vi "UPDATE ITEMS.vi"(10 "DATA IN":T3, 11 "connection reference in":T1) -> (3 "connection reference out":T1)   [LabVIEW 2019]
uses:
  Controls/Table Data Types/Inventory Data Type.ctl
  <vilib>/addons/database/Connection.llb/Conn ObjectReference.ctl
  Controls/Column Names/Inventory Column Names.ctl
  <vilib>/addons/database/NI_Database_API.lvlib
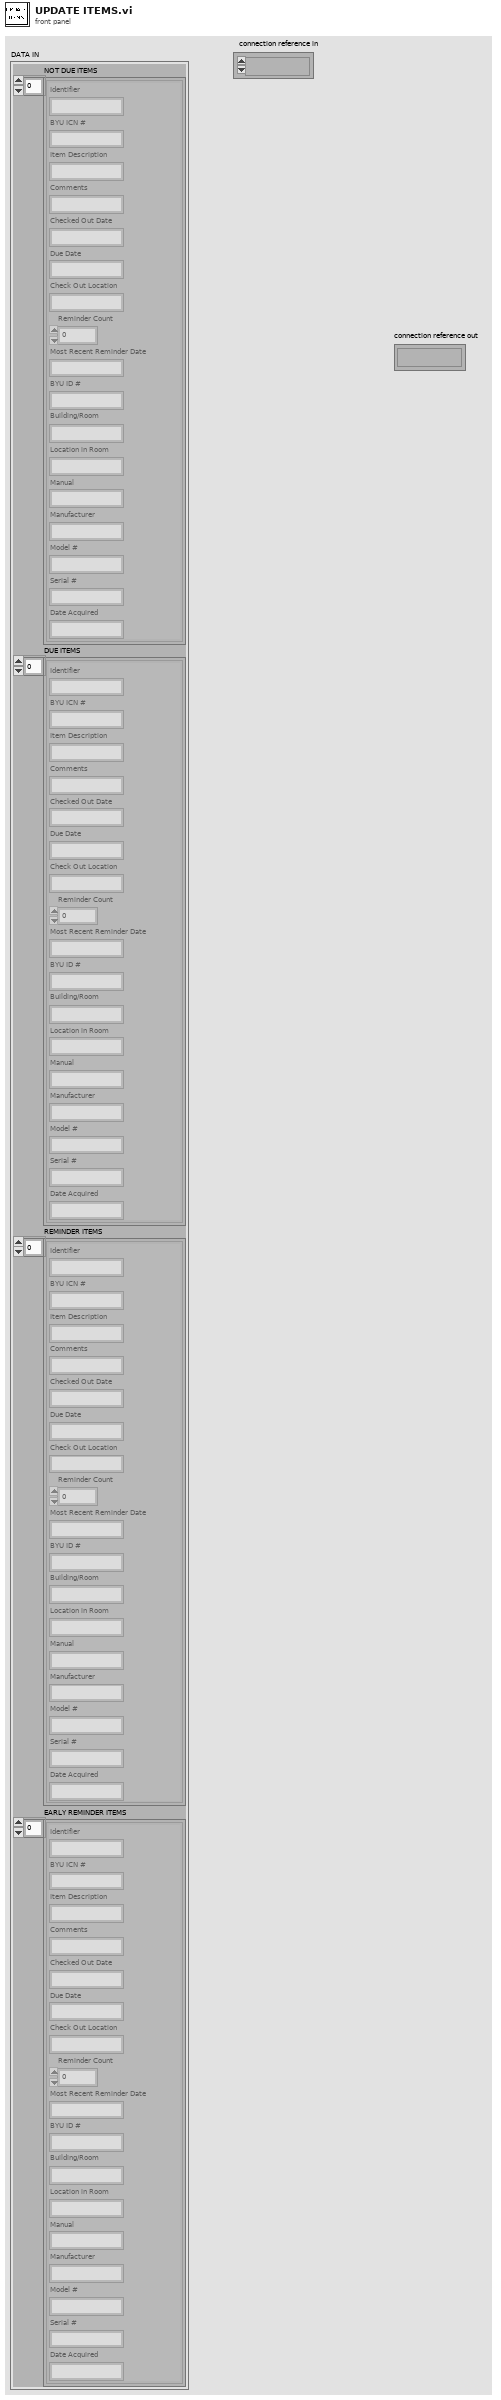
[diagram p1: front panel]
types:
  T1 = typedef "NI_Database_API.lvlib/Conn ObjectReference.ctl" = refnum<k1>
  T2 = typedef "Inventory Data Type.ctl" = cluster{"Identifier":string, "BYU ICN #":string, "Item Description":string, "Comments":string, "Checked Out Date":string, "Due Date":string, "Check Out Location":string, "Reminder Count":i32, "Most Recent Reminder Date":string, "BYU ID #":string, "Building/Room":string, "Location in Room":string, "Manual":string, "Manufacturer":string, "Model #":string, "Serial #":string, "Date Acquired":string}
  T3 = cluster{"NOT DUE ITEMS":T2[], "DUE ITEMS":T2[], "REMINDER ITEMS":T2[], "EARLY REMINDER ITEMS":T2[]}
  T4 = typedef "Inventory Column Names.ctl" = string[]
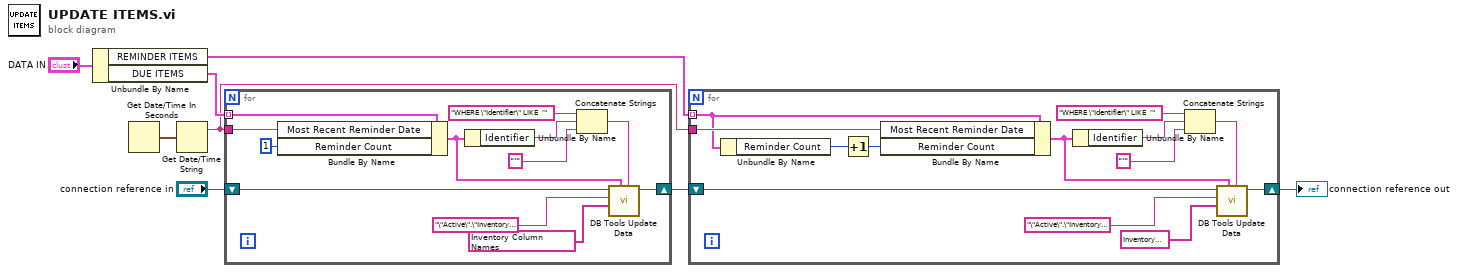
[diagram p0: block diagram]
diagram:
  n1 = Unbundle By Name("DATA IN") -> ("REMINDER ITEMS"=w3:T2[], "DUE ITEMS"=w7:T2[])
  n2 = Get Date/Time In Seconds() -> (seconds since 1Jan1904=w6:timestamp)
  n3 = Get Date/Time String(seconds (now)=w6) -> (date string=w2:string)  [unwired: 2 in, 1 out]
  n4 = for {
    tunnel: w7 -> [w20] mode=indexing
    tunnel: w2 -> [w18]
    shift-right: [w9] -> w4
    shift-left: "connection reference in" -> [w12]
    n5 = Bundle By Name(cluster=w20, "Most Recent Reminder Date"=w18, "Reminder Count"=1) -> (w13:T2)
    n6 = Unbundle By Name(w13) -> ("Identifier"=w16:string)
    n7 = Concatenate Strings("WHERE \"Identifier\" LIKE  '", w16, "'") -> (w14:string)
    n8 = call <vilib>:"DB Tools Update Data.vi"("condition"=w14, "data"=w13, "columns"=T4 ["\"Identifier\"", "\"BYU ICN #\"", "\"Item Description\"", "\"Comments\"", "\"Checked Out Date\"", "\"Due Date\"", "\"Check Out Location\"", "\"Reminder Count\"", "\"Most Recent Reminder Date\"", "\"BYU ID #\"", "\"Building/Room\"", "\"Location in Room\"", "\"Manual\"", "\"Manufacturer\"", "\"Model #\"", "\"Serial #\"", "\"Date Acquired\""] ("INVENTORY COLUMN NAMES"), "table"="\"Active\".\"Inventory\"", "connection reference"=w12) -> ("connection reference out"=w9:T1)  [unwired: 5 in, 1 out]
  }
  n9 = for {
    tunnel: w3 -> [w23] mode=indexing
    tunnel: w2 -> [w33]
    shift-right: [w24] -> w1
    shift-left: w4 -> [w27]
    n10 = Unbundle By Name(w23) -> ("Reminder Count"=w22:i32)
    n11 = Increment(x=w22) -> (x+1=w21:i32)
    n12 = Bundle By Name(cluster=w23, "Most Recent Reminder Date"=w33, "Reminder Count"=w21) -> (w28:T2)
    n13 = Unbundle By Name(w28) -> ("Identifier"=w31:string)
    n14 = Concatenate Strings("WHERE \"Identifier\" LIKE  '", w31, "'") -> (w29:string)
    n15 = call <vilib>:"DB Tools Update Data.vi"("condition"=w29, "data"=w28, "columns"=T4 ["\"Identifier\"", "\"BYU ICN #\"", "\"Item Description\"", "\"Comments\"", "\"Checked Out Date\"", "\"Due Date\"", "\"Check Out Location\"", "\"Reminder Count\"", "\"Most Recent Reminder Date\"", "\"BYU ID #\"", "\"Building/Room\"", "\"Location in Room\"", "\"Manual\"", "\"Manufacturer\"", "\"Model #\"", "\"Serial #\"", "\"Date Acquired\""] ("INVENTORY COLUMN NAMES"), "table"="\"Active\".\"Inventory\"", "connection reference"=w27) -> ("connection reference out"=w24:T1)  [unwired: 5 in, 1 out]
  }
  "connection reference out" <- w1
